vi "Create Subpanel (by ref).vi"(5 "Scrollbars (off)":T1, 7 "Sizing":T2, 8 "error in":errorcluster, 10 "Subpanel Ref":refnum<vi>, 11 "UI VI Reference (caller)":refnum<vi>) -> (0 "error out":errorcluster, 3 "Flex Subpanel out":refnum<class "Flex UI Subpanel.lvclass">)   [LabVIEW 2016, in "Flex UI Subpanel.lvclass"]
uses:
  Flex UI Subpanel.lvclass
  C:/VI Packages/Flex UI/Flex UI (Parent)/Flex UI.lvclass
  Enum - Sizing.ctl
  Cluster - Scrollbar Visibility.ctl
  Flex UI (Parent)/Flex UI.lvclass/Flex UI.ctl
  Flex UI Subpanel.lvclass/Flex UI Subpanel.ctl
  Flex UI (Parent)/Flex UI.lvclass
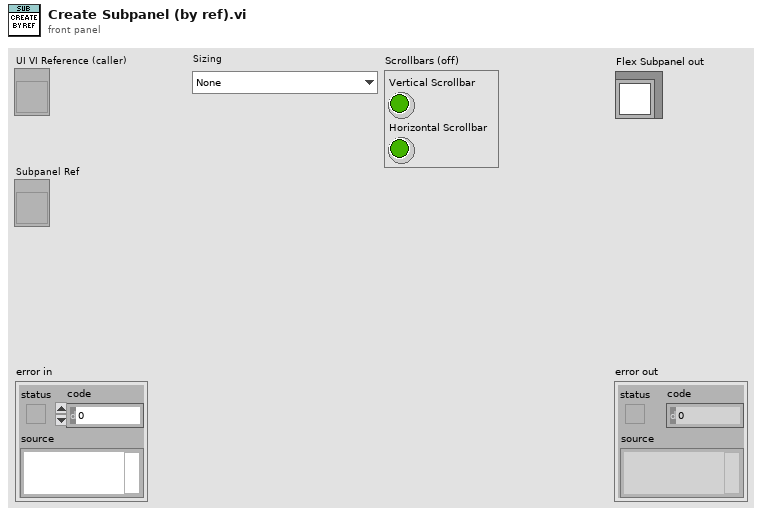
[diagram p1: front panel]
types:
  T1 = typedef "Flex UI Subpanel.lvclass/Cluster - Scrollbar Visibility.ctl" = cluster{"Vertical Scrollbar":bool, "Horizontal Scrollbar":bool}
  T2 = typedef "Flex UI Subpanel.lvclass/Enum - Sizing.ctl" = enum16{"None", "Largest Decoration", "Maximize"}
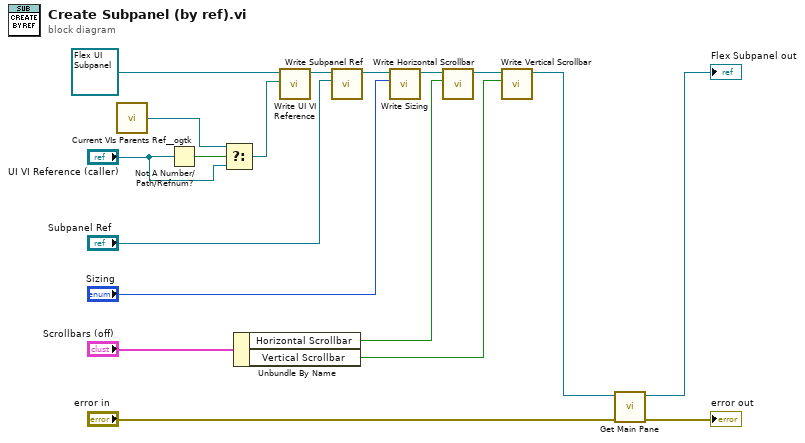
[diagram p0: block diagram]
diagram:
  n1 = call <userlib>:"Current VIs Parents Ref__ogtk.vi"() -> ("Calling VI's Reference"=w16:refnum<vi>)  [unwired: 2 in]
  n2 = Not A Number/Path/Refnum?(number/path/refnum="UI VI Reference (caller)") -> (NaN/Path/Refnum?=w17:bool)
  n3 = Select(t=w16, s=w17, f="UI VI Reference (caller)") -> (s? t:f=w15:refnum<vi>)
  n4 = Unbundle By Name("Scrollbars (off)") -> ("Horizontal Scrollbar"=w5:bool, "Vertical Scrollbar"=w4:bool)
  n5 = call "Write UI VI Reference.vi"("UI VI Reference"=w15, "Flex UI in"=refnum<class "Flex UI Subpanel.lvclass"> refnum ("Flex Subpanel out")) -> ("Flex UI out"=w12:refnum<class "Flex UI Subpanel.lvclass">)  [unwired: 9 in]
  n6 = call "Write Subpanel Ref.vi"("Subpanel Ref"="Subpanel Ref", "Flex Subpanel in"=w12) -> ("Flex Subpanel out"=w11:refnum<class "Flex UI Subpanel.lvclass">)  [unwired: 9 in]
  n7 = call "Write Sizing.vi"("Sizing"="Sizing", "Flex Subpanel in"=w11) -> ("Flex Subpanel out"=w9:refnum<class "Flex UI Subpanel.lvclass">)  [unwired: 9 in]
  n8 = call "Write Horizontal Scrollbar.vi"("Horizontal Scrollbar"=w5, "Flex Subpanel in"=w9) -> ("Flex Subpanel out"=w7:refnum<class "Flex UI Subpanel.lvclass">)  [unwired: 9 in]
  n9 = call "Write Vertical Scrollbar.vi"("Vertical Scrollbar"=w4, "Flex Subpanel in"=w7) -> ("Flex Subpanel out"=w2:refnum<class "Flex UI Subpanel.lvclass">)  [unwired: 9 in]
  n10 = call-dynamic "Get Main Pane.vi"("error in"="error in", "Flex UI in"=w2) -> ("error out"=→"error out":errorcluster, "Flex UI out"=→"Flex Subpanel out":refnum<class "Flex UI Subpanel.lvclass">)  [unwired: 8 in]
